vi "write_roi_command.vi"(10 "ROI Max":dbl, 11 "ROI Min":dbl) -> (2 "Command Out":string)   [LabVIEW 2015]
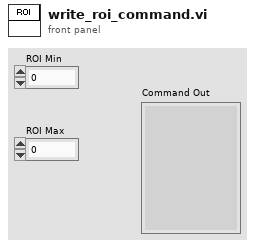
[diagram p1: front panel]
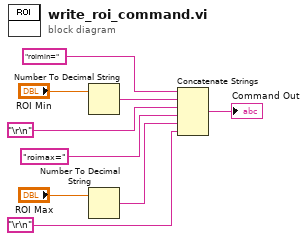
[diagram p0: block diagram]
diagram:
  n1 = Number To Decimal String(number="ROI Min") -> (decimal integer string=w7:string)  [unwired: 1 in]
  n2 = Number To Decimal String(number="ROI Max") -> (decimal integer string=w4:string)  [unwired: 1 in]
  n3 = Concatenate Strings("roimin=", w7, "\r\n", "roimax=", w4, "\r\n") -> (→"Command Out":string)
